vi "pattern.vi"(0 "Error In":errorcluster, 1 "Numeric":i32) -> (2 "Error Out":errorcluster, 3 "Pattern":i16[](graph), 4 "Pattern 2":i16[](graph))   [LabVIEW 2014]
uses:
  wlmData.dll
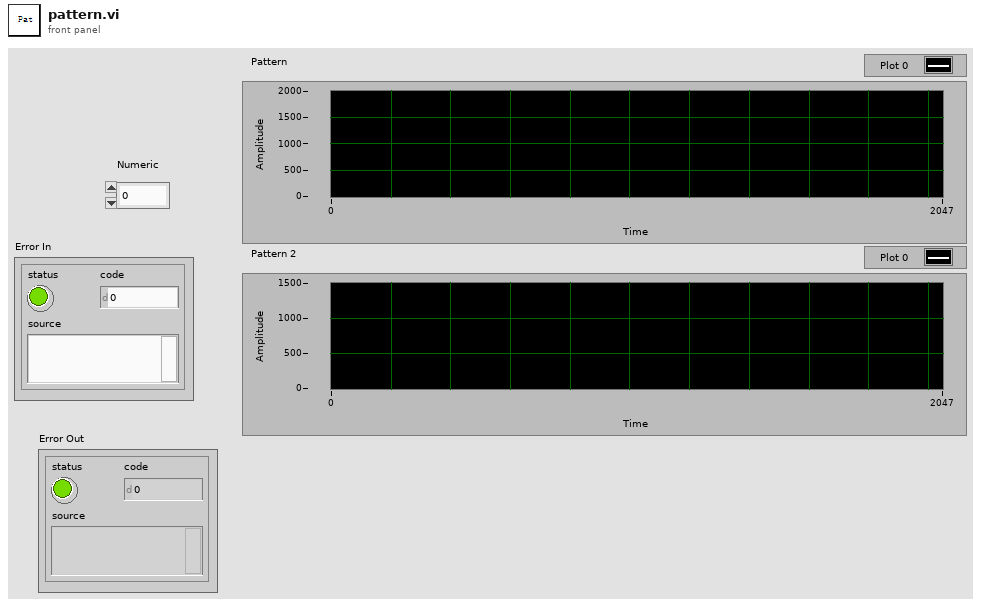
[diagram p1: front panel]
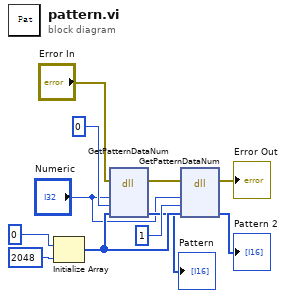
[diagram p0: block diagram]
diagram:
  n1 = Initialize Array(0, 2048 ("dimension size")) -> (w7:i32[])
  n2 = dll-call lib="wlmData.dll" fn="GetPatternDataNum"(error in="Error In", "channel"="Numeric", "Index"=0, "array"=w7) -> (error out=w8:errorcluster, "array"=→"Pattern":i16[])  [unwired: 5 in, 1 out]
  n3 = dll-call lib="wlmData.dll" fn="GetPatternDataNum"(error in=w8, "channel"="Numeric", "Index"=1, "array"=w7) -> (error out=→"Error Out":errorcluster, "array"=→"Pattern 2":i16[])  [unwired: 5 in, 1 out]
